vi "PH_Img_BaseClass.get i attribute.vi"(0 "i ref in":refnum<vi>, 5 "error in (no error)":errorcluster) -> (14 "i ref out":refnum<vi>, 16 "i attribute":T1={"GUI Refs"={"Timeout"=refnum, "Image"=refnum, "Palette"=refnum, "Timeout Set"=refnum}, "Timeout Image [ms]"=1000, "Default Periodic Period [ms]"=0, "Camera"={"Instancename"="", "Notifier"=refnum}, "Palette"=0, "Cam Settings"={"Cam ID"="", "Gain"=0.0, "Brightness"=0.0, "Shutter"=0.0, "Cam Info Failure"=FALSE, "Mode"=0}} {"Palette" items=["Grey", "Binary", "Gradient", "Rainbow", "Temperature"]}, 19 "error out":errorcluster)   [LabVIEW 2014, in "PH_Img_BaseClass.lvlib"]
doc: "Gets the i attribute data of an object.\n\nLicense Agreement for this software:\n\nCopyright (C)\nGesellschaft für Schwerionenforschung, GSI\nPlanckstr. 1\n64291 Darmstadt\nGermany\n\nContact: D.Beck@gsi.de \n\nThis program is free software; you can redistribute it and/or modify it under the terms of the GNU General Public License as published by the Free Software Foundation; either version 2 of the license, or (at your option) any later version.\n\nThis program is distributed in the hope that it will be useful, but WITHOUT ANY WARRANTY; without even the implied warranty of MERCHANTABILITY or FITNESS FOR A PARTICULAR PURPOSE. See the GNU General License for more details (http://www.gnu.org).\n\nGesellschaft für Schwerionenforschung, GSI\nPlanckstr. 1, 64291 Darmstadt, Germany\nFor all questions and ideas contact: M.Richter@gsi.de, H.Brand@gsi.de or D.Beck@gsi.de.\nLast update: 17-JUN-2004"
uses:
  PH_Img_BaseClass.lvlib
  PH_Img_BaseClass.i attribute.ctl
  PH_Img_BaseClass.GUI Refs.ctl
  PH_Img_BaseClass.Palette.ctl
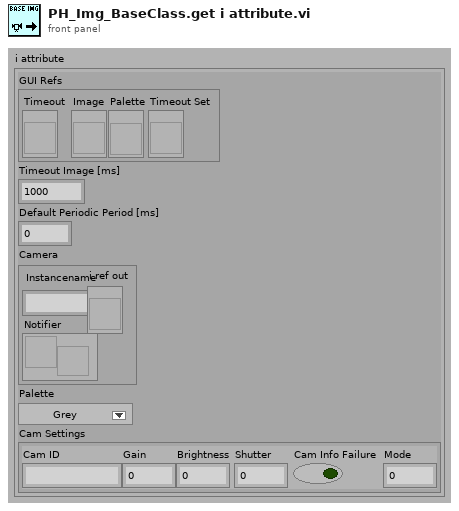
[diagram p1: front panel]
types:
  T1 = typedef "PH_Img_BaseClass.lvlib/PH_Img_BaseClass.i attribute.ctl" = cluster{"GUI Refs":T2, "Timeout Image [ms]":i32, "Default Periodic Period [ms]":i32, "Camera":cluster{"Instancename":string, "Notifier":refnum<notifier>}, "Palette":T3, "Cam Settings":cluster{"Cam ID":string, "Gain":dbl, "Brightness":dbl, "Shutter":dbl, "Cam Info Failure":bool, "Mode":i32}}
  T2 = typedef "PH_Img_BaseClass.lvlib/PH_Img_BaseClass.GUI Refs.ctl" = cluster{"Timeout":refnum<vi>, "Image":refnum<vi>, "Palette":refnum<vi>, "Timeout Set":refnum<vi>}
  T3 = typedef "PH_Img_BaseClass.lvlib/PH_Img_BaseClass.Palette.ctl" = i32
  T4 = enum16{"SetAttribute", "GetAttribute", "CreateAttribute", "DestroyAttribute", "DestroyAllAtributes"}
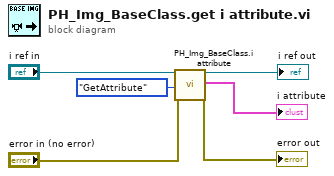
[diagram p0: block diagram]
diagram:
  n1 = call "PH_Img_BaseClass.i attribute.vi"("VI Refnum"="i ref in", "Action"=T4."GetAttribute", "error in (no error)"="error in (no error)") -> ("VI Refnum out"=→"i ref out":refnum<vi>, "CLASS.i attribute out"=→"i attribute":T1, "error out"=→"error out":errorcluster)  [unwired: 14 in]
